vi "Send Frame.vi"(8 "error in (no error)":errorcluster, 10 "Data in":T1 {"Measurements and statistics"."Running, perc. of time" format="%05.2f"}) -> (0 "error out":errorcluster)   [LabVIEW 2018, in "Stream Data.lvlib"]
doc: "Requests to send a single data frame.\n_____\nCreated using Delacor QMH Event Scripter 4.2.1.88."
uses:
  Stream Data.lvlib
  SubVi's/Controls/CTL_Full_data_frame.ctl
  SubVi's/Controls/CTL_Animal_Coordinates_and_Speed.ctl
  SubVi's/Controls/CTL_Measurements_and_Statistics.ctl
  Send Frame Argument--cluster.ctl
  Common_Resources.lvlib
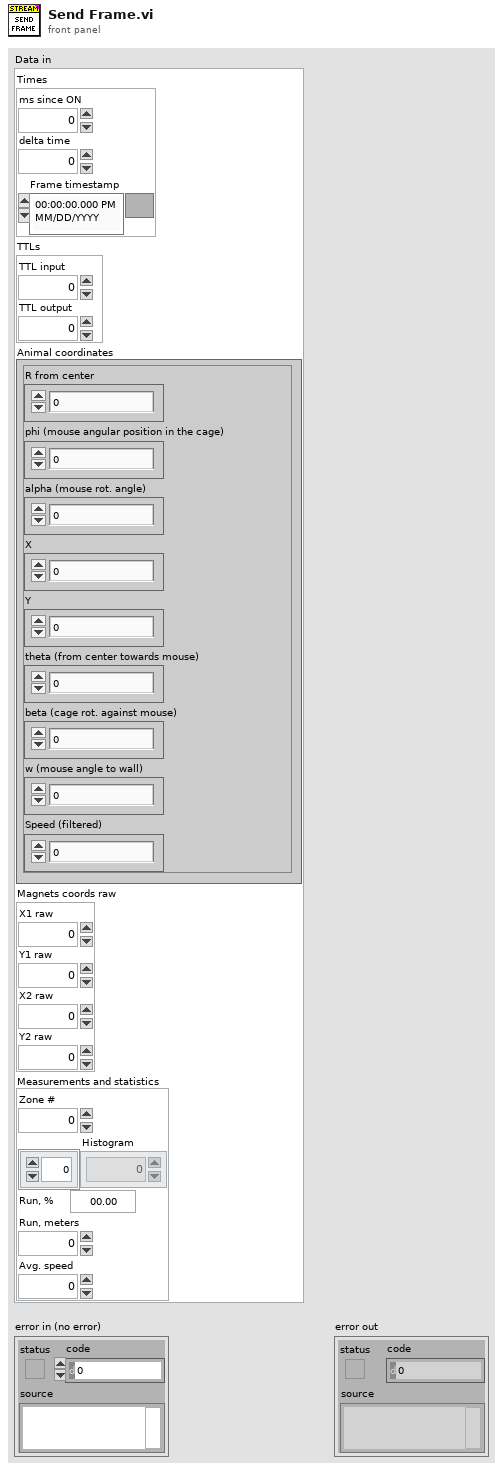
[diagram p1: front panel]
types:
  T1 = typedef "Common_Resources.lvlib/CTL_Full_data_frame.ctl" = cluster{"Times":cluster{"ms since ON":u32, "delta time":u32, "Frame timestamp":timestamp}, "TTLs":cluster{"TTL input":i16, "TTL output":i16}, "Animal coordinates":T2, "Magnets coords raw":cluster{"X1 raw":dbl, "Y1 raw":dbl, "X2 raw":dbl, "Y2 raw":dbl}, "Measurements and statistics":T3}
  T2 = typedef "Common_Resources.lvlib/CTL_Animal_Coordinates_and_Speed.ctl" = cluster{"R from center":dbl, "phi (mouse angular position in the cage)":dbl, "alpha (mouse rot. angle)":dbl, "X":dbl, "Y":dbl, "theta (from center towards mouse)":dbl, "beta (cage rot. against mouse)":dbl, "w (mouse angle to wall)":dbl, "Speed (filtered)":dbl}
  T3 = typedef "Common_Resources.lvlib/CTL_Measurements_and_Statistics.ctl" = cluster{"Zone #":i8, "Histogram":dbl[], "Running, perc. of time":dbl, "Run, meters":dbl, "Avg. speed":dbl}
  T4 = typedef "Stream Data.lvlib/Send Frame Argument--cluster.ctl" = cluster{"Data in":T1}
  T5 = typedef "Stream Data.lvlib/Request Events--cluster.ctl" = cluster{"Stop Module":refnum<user-event>, "Show Panel":refnum<user-event>, "Hide Panel":refnum<user-event>, "Get Module Execution Status":refnum<user-event>, "Show Diagram":refnum<user-event>, "Send Frame":refnum<user-event>, "Open Serial Port":refnum<user-event>, "Change Serial Port":refnum<user-event>, "Close Serial Port":refnum<user-event>, "Update Status":refnum<user-event>, "Prepare to Exit":refnum<user-event>}
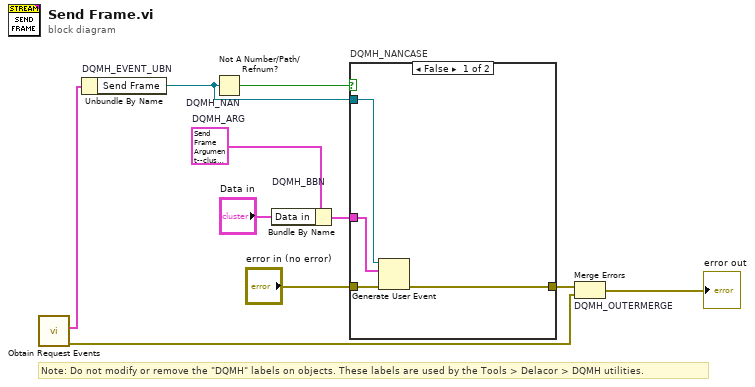
[diagram p0: block diagram]
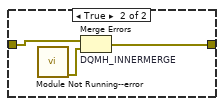
[diagram p2: hidden frame]
diagram:
  w4 = T4 {"Data in"={"Times"={"ms since ON"=0, "delta time"=0, "Frame timestamp"=timestamp(0 s since 1904-01-01)}, "TTLs"={"TTL input"=0, "TTL output"=0}, "Animal coordinates"={"R from center"=0.0, "phi (mouse angular position in the cage)"=0.0, "alpha (mouse rot. angle)"=0.0, "X"=0.0, "Y"=0.0, "theta (from center towards mouse)"=0.0, "beta (cage rot. against mouse)"=0.0, "w (mouse angle to wall)"=0.0, "Speed (filtered)"=0.0}, "Magnets coords raw"={"X1 raw"=0.0, "Y1 raw"=0.0, "X2 raw"=0.0, "Y2 raw"=0.0}, "Measurements and statistics"={"Zone #"=0, "Histogram"=[], "Running, perc. of time"=0.0, "Run, meters"=0.0, "Avg. speed"=0.0}}}  # DQMH_ARG
  # "Note: Do not modify or remove the \"DQMH\" labels on objects. These labels are used by the Tools > Delacor > DQMH utilities."
  n1 = call "Obtain Request Events.vi"() -> ("error out"=w2:errorcluster, "Stream Data Request Events"=w1:T5)  [unwired: 10 in]
  n2 = Unbundle By Name "DQMH_EVENT_UBN"(w1) -> ("Send Frame"=w6:refnum<user-event>)
  n3 = Not A Number/Path/Refnum? "DQMH_NAN"(number/path/refnum=w6) -> (NaN/Path/Refnum?=w7:bool)
  n4 = Bundle By Name "DQMH_BBN"(cluster=w4, "Data in"="Data in") -> (w8:T4)
  n5 = case "DQMH_NANCASE" shown="False" w7 {
    tunnel: "error in (no error)" -> [w14 w17]
    tunnel: [w13 w16] -> w5
    tunnel: w6 -> [w12 _]
    tunnel: w8 -> [w11 _]
    frame False {
      n6 = Generate User Event(user event=w12, event data cluster=w11, error in=w14) -> (error out=w13:errorcluster)  [unwired: 1 in, 1 out]
    }
    frame True {
      n7 = call "Module Not Running--error.vi"() -> ("error out"=w15:errorcluster)  [unwired: 11 in]
      n8 = Merge Errors "DQMH_INNERMERGE"(w17, w15) -> (w16:errorcluster)
    }
  }
  n9 = Merge Errors "DQMH_OUTERMERGE"(w5, w2) -> (→"error out":errorcluster)
